vi "ROS_Topic_Write_Stop_Continuous_Primitive.vi"() -> ()   [LabVIEW 2010]
doc: "Instructs the server to stop publishing messages continuously."
uses:
  <userlib>/ROSforLV_0.1/ROS/Code/SubVIs/_ROSControl.ctl
  <userlib>/ROSforLV_0.1/ROS/Code/SubVIs/_ROSDirection.ctl
panel:
  in  "ROS in":T1
  out "ROS out":T1
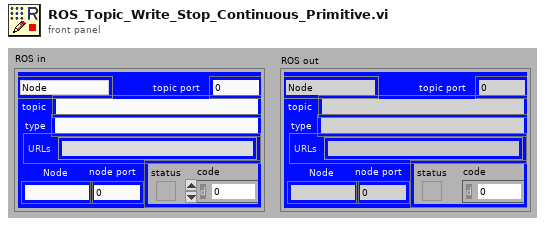
[diagram p1: front panel]
types:
  T1 = typedef "_ROSControl.ctl" = cluster{"topic port":u16, "Node":string, "topic":string, "type":string, "node port":u32, "error ":errorcluster, "Direction":T2, "APIs":string[]}
  T2 = typedef "_ROSDirection.ctl" = enum16{"Node", "Publisher", "Subscriber", "Service Client"}
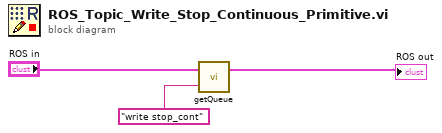
[diagram p0: block diagram]
diagram:
  n1 = call <userlib>:"getQueue.vi"("queue msg"="write stop_cont" ("t"), "ROS in"="ROS in") -> ("ROS out"=→"ROS out":T1)  [unwired: 1 in]
